vi "Set BC.vi"(8 "error in (no error)":errorcluster, 10 "BC":variant, 11 "BC_Evolut_2D_Numeric in":refnum<class "NI_BC_Evolut_2D_Numeric.lvclass">) -> (0 "error out":errorcluster, 3 "BC_Evolut_2D_Numeric out":refnum<class "NI_BC_Evolut_2D_Numeric.lvclass">)   [LabVIEW 2017, in "NI_PDE.lvlib" / "NI_BC_Evolut_2D_Numeric.lvclass"]
uses:
  <vilib>/gmath/pde.llb/BCClass/BC_Evolut_2D_Numeric/NI_BC_Evolut_2D_Numeric.lvclass
  <vilib>/gmath/pde.llb/BCClass/BC_Evolut_2D_Numeric/BC Data.ctl
  <vilib>/gmath/pde.llb/Common/PDE_BC Type.ctl
  <vilib>/gmath/pde.llb/Common/PDE_BC Position 2D.ctl
  <vilib>/gmath/pde.llb/BCClass/BC_Evolut_2D_Numeric/NI_BC_Evolut_2D_Numeric.lvclass/NI_BC_Evolut_2D_Numeric.ctl
  <vilib>/gmath/NI_PDE.lvlib
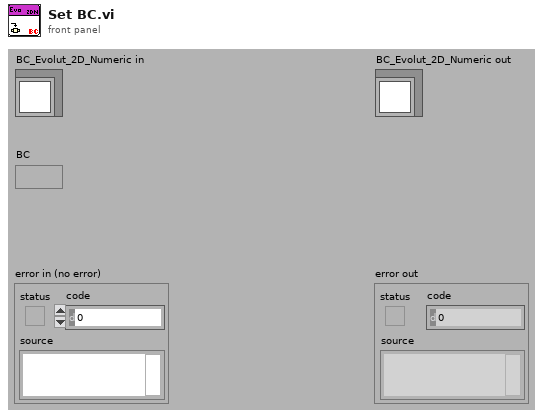
[diagram p1: front panel]
types:
  T1 = typedef "NI_PDE.lvlib/NI_BC_Evolut_2D_Numeric.lvclass/BC Data.ctl" = cluster{"type":T2, "position":T3, "G":dbl[][]}
  T2 = typedef "NI_PDE.lvlib/PDE_BC Type.ctl" = i32
  T3 = typedef "NI_PDE.lvlib/PDE_BC Position 2D.ctl" = i32
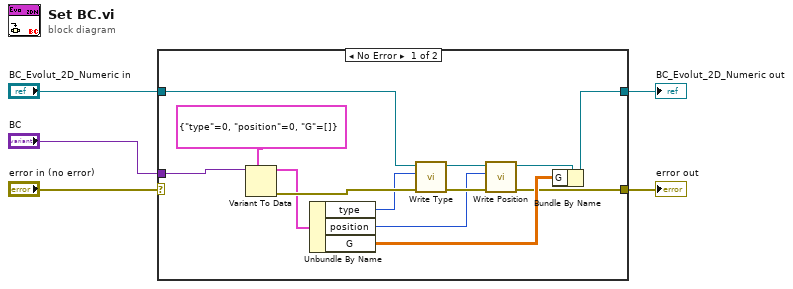
[diagram p0: block diagram]
diagram:
  n1 = case shown="No Error" "error in (no error)" {
    selector: "error in (no error)" -> [_ w20]
    tunnel: "BC_Evolut_2D_Numeric in" -> [w15 w19]
    tunnel: [w8 w19] -> w5
    tunnel: [w6 w20] -> w4
    tunnel: "BC" -> [w10 _]
    frame No Error {
      n2 = Variant To Data(type=T1 {"type"=0, "position"=0, "G"=[]} ("BC data"), Variant=w10) -> (data=w13:T1, error out=w14:errorcluster)  [unwired: 1 in]
      n3 = Unbundle By Name(w13) -> ("type"=w12:T2, "position"=w11:T3, "G"=w7:dbl[][])
      n4 = call-dynamic "Write Type.vi"("error in (no error)"=w14, "BC type"=w12, "BC.lvclass in"=w15) -> ("error out"=w16:errorcluster, "BC.lvclass out"=w17:refnum<class "NI_BC_Evolut_2D_Numeric.lvclass">)  [unwired: 7 out]
      n5 = call-dynamic "Write Position.vi"("error in (no error)"=w16, "BC position 2D"=w11, "BC_Evolut_2D.lvclass in"=w17) -> ("error out"=w6:errorcluster, "BC_Evolut_2D.lvclass out"=w9:refnum<class "NI_BC_Evolut_2D_Numeric.lvclass">)  [unwired: 7 out]
      n6 = Bundle By Name(cluster=w9, "G"=w7) -> (w8:refnum<class "NI_BC_Evolut_2D_Numeric.lvclass">)
    }
    frame Error {
    }
  }
  "BC_Evolut_2D_Numeric out" <- w5
  "error out" <- w4
